vi "Master Data Handler.vi"(0 "transfer settings":T2 {"Direction Change Bit" max=64 step=1; "Transfer Length (bits)" min=1 max=64 step=1}, 9 "controller interface":T1) -> (4 "shift MOSI":bool, 6 "sample MISO":bool, 8 "dir change":bool, 10 "read pending":bool, 15 "done":bool)   [LabVIEW 2014, in "NI SPI IP (FPGA).lvlib"]
doc: "This VI creates control signals to shift in MISO data and shift out MOSI data as well as determining when a transaction has completed."
uses:
  <userlib>/_NI SPI IP/FPGA/Controllers/NI SPI IP (FPGA).lvlib
  <userlib>/_NI SPI IP/FPGA/Controllers/Public/Transfer Settings.ctl
  <userlib>/_NI SPI IP/FPGA/Controllers/Private/Controller Interface.ctl
panel:
  # "This VI creates control signals to shift in MISO data and shift out MOSI data as well as determining when a transaction has completed."
  # "Controller interface cluster is simply a group of controls from the main SPI state machine. These controls are clustered for ease of use."
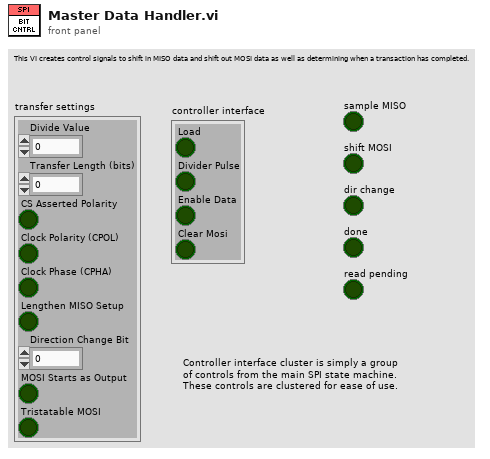
[diagram p1: front panel]
types:
  T1 = typedef "NI SPI IP (FPGA).lvlib/Controller Interface.ctl" = cluster{"Load":bool, "Divider Pulse":bool, "Enable Data":bool, "Clear Mosi":bool}
  T2 = typedef "NI SPI IP (FPGA).lvlib/Transfer Settings.ctl" = cluster{"Divide Value":u8, "Transfer Length (bits)":u8, "CS Asserted Polarity":bool, "Clock Polarity (CPOL)":bool, "Clock Phase (CPHA)":bool, "Lengthen MISO Setup":bool, "Direction Change Bit":u8, "MOSI Starts as Output":bool, "Tristatable MOSI":bool}
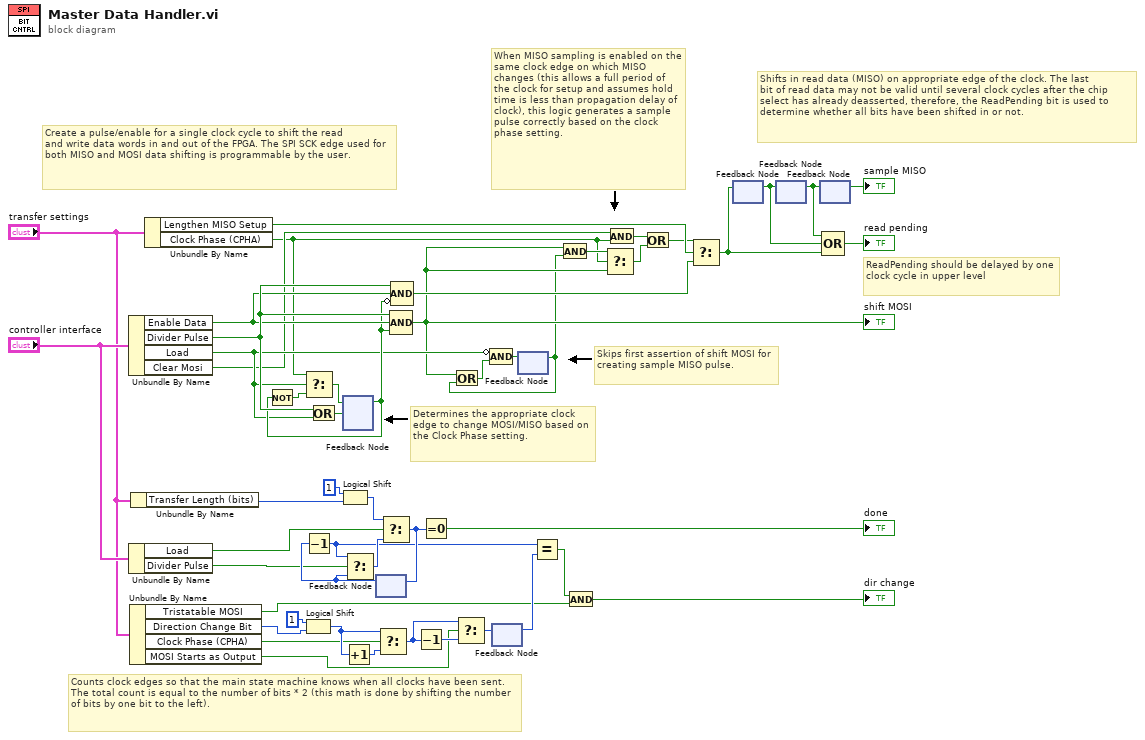
[diagram p0: block diagram]
diagram:
  # "Skips first assertion of shift MOSI for creating sample MISO pulse."
  # "When MISO sampling is enabled on the same clock edge on which MISO changes (this allows a full period of the clock for setup and assumes hold time is less than propagation delay of clock), this logic generates a sample pulse correctly based on the clock phase setting."
  # "Determines the appropriate clock edge to change MOSI/MISO based on the Clock Phase setting."
  # "Counts clock edges so that the main state machine knows when all clocks have been sent. The total count is equal to the number of bits * 2 (this math is done by shifting the number of bits by one bit to the left)."
  # "Create a pulse/enable for a single clock cycle to shift the read\nand write data words in and out of the FPGA. The SPI SCK edge used for both MISO and MOSI data shifting is programmable by the user."
  # "Shifts in read data (MISO) on appropriate edge of the clock. The last\nbit of read data may not be valid until several clock cycles after the chip select has already deasserted, therefore, the ReadPending bit is used to determine whether all bits have been shifted in or not."
  # "ReadPending should be delayed by one clock cycle in upper level"
  n1 = Unbundle By Name("controller interface") -> ("Enable Data"=w31:bool, "Divider Pulse"=w32:bool, "Load"=w23:bool, "Clear Mosi"=w22:bool)
  n2 = Unbundle By Name("controller interface") -> ("Load"=w43:bool, "Divider Pulse"=w44:bool)
  n3 = Unbundle By Name("transfer settings") -> ("Tristatable MOSI"=w4:bool, "Direction Change Bit"=w10:u8, "Clock Phase (CPHA)"=w12:bool, "MOSI Starts as Output"=w6:bool)
  n4 = Unbundle By Name("transfer settings") -> ("Transfer Length (bits)"=w37:u8)
  n5 = Unbundle By Name("transfer settings") -> ("Lengthen MISO Setup"=w29:bool, "Clock Phase (CPHA)"=w21:bool)
  n6 = Logical Shift(y=i8 1, x=w10) -> (x << y=w15:u8)
  n7 = Or(x=w32, y=w23) -> (x .or. y?=w35:bool)
  n8 = Logical Shift(y=i8 1, x=w37) -> (x << y=w47:u8)
  n9 = feedback #1() -> (w30:bool)  [unwired: 1 in]
  n10 = Not(x=w30) -> (.not. x?=w33:bool)
  n11 = Select(t=w21, s=w23, f=w33) -> (s? t:f=w34:bool)
  n12 = feedback-in #1(w34, w35) -> ()
  n13 = Increment(x=w15) -> (x+1=w14:u8)
  n14 = feedback #2() -> (w48:u8)  [unwired: 1 in]
  n15 = Decrement(x=w48) -> (x-1=w17:u8)
  n16 = Select(t=w17, s=w44, f=w48) -> (s? t:f=w46:u8)
  n17 = Select(t=w15, s=w12, f=w14) -> (s? t:f=w8:u8)
  n18 = Select(t=w47, s=w43, f=w46) -> (s? t:f=w18:u8)
  n19 = feedback-in #2(w18) -> ()
  n20 = Compound Arithmetic op=AND(w32, w31, w30) -> (w2:bool)
  "shift MOSI" <- w2
  n21 = Compound Arithmetic op=AND(w32, w31, invert w30) -> (w28:bool)
  n22 = Decrement(x=w8) -> (x-1=w9:u8)
  n23 = Equal To 0?(x=w18) -> (x = 0?=→"done":bool)
  n24 = Select(t=w8, s=w6, f=w9) -> (s? t:f=w7:u8)
  n25 = feedback #3() -> (w13:u8)  [unwired: 1 in]
  n26 = feedback-in #3(w7) -> ()
  n27 = feedback #4() -> (w1:bool)  [unwired: 1 in]
  n28 = Or(x=w2, y=w1) -> (x .or. y?=w39:bool)
  n29 = Compound Arithmetic op=AND(invert w23, w39) -> (w38:bool)
  n30 = feedback-in #4(w38) -> ()
  n31 = Equal?(x=w17, y=w13) -> (x = y?=w5:bool)
  n32 = And(x=w2, y=w1) -> (x .and. y?=w25:bool)
  n33 = And(x=w5, y=w4) -> (x .and. y?=→"dir change":bool)
  n34 = Select(t=w25, s=w21, f=w2) -> (s? t:f=w24:bool)
  n35 = And(x=w22, y=w21) -> (x .and. y?=w20:bool)
  n36 = Or(x=w20, y=w24) -> (x .or. y?=w26:bool)
  n37 = Select(t=w26, s=w29, f=w28) -> (s? t:f=w27:bool)
  n38 = feedback #5() -> (w40:bool)  [unwired: 1 in]
  n39 = feedback-in #5(w27) -> ()
  n40 = feedback #6() -> (w41:bool)  [unwired: 1 in]
  n41 = feedback-in #6(w40) -> ()
  n42 = feedback #7() -> (→"sample MISO":bool)  [unwired: 1 in]
  n43 = feedback-in #7(w41) -> ()
  n44 = Compound Arithmetic op=OR(w41, w40, w27) -> (→"read pending":bool)
